vi "WPI_DashboardConvert to Log Format.vi"(11 "Frequent DB Data":T1) -> (3 "Logged Data":T2)   [LabVIEW 2017]
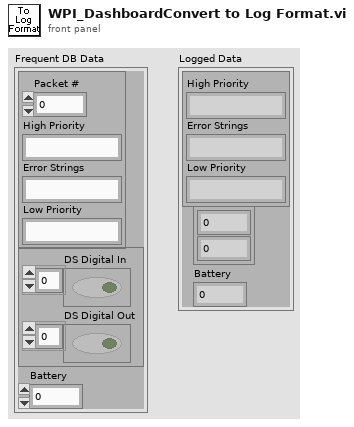
[diagram p1: front panel]
types:
  T1 = cluster{cluster{"Packet #":u8, "High Priority":string, "Error Strings":string, "Low Priority":string}, cluster{"DS Digital In":bool[], "DS Digital Out":bool[]}, "Battery":sgl}
  T2 = cluster{cluster{"High Priority":string, "Error Strings":string, "Low Priority":string}, cluster{u8, u8}, "Battery":sgl}
  T3 = cluster{"Packet #":u8, "High Priority":string, "Error Strings":string, "Low Priority":string}
  T4 = cluster{"DS Digital In":bool[], "DS Digital Out":bool[]}
  T5 = cluster{"High Priority":string, "Error Strings":string, "Low Priority":string}
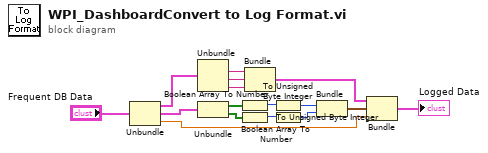
[diagram p0: block diagram]
diagram:
  n1 = Unbundle("Frequent DB Data") -> (w12:T3, w1:T4, "Battery"=w10:sgl)
  n2 = Unbundle(w12) -> ("High Priority"=w13:string, "Error Strings"=w15:string, "Low Priority"=w14:string)  [unwired: 1 out]
  n3 = Unbundle(w1) -> ("DS Digital In"=w2:bool[], "DS Digital Out"=w6:bool[])
  n4 = Boolean Array To Number(Boolean array=w2) -> (number=w3:u32)
  n5 = Boolean Array To Number(Boolean array=w6) -> (number=w5:u32)
  n6 = Bundle("High Priority"=w13, "Error Strings"=w15, "Low Priority"=w14) -> (w16:T5)  [unwired: 1 in]
  n7 = To Unsigned Byte Integer(number=w3) -> (unsigned 8bit integer=w4:u8)
  n8 = To Unsigned Byte Integer(number=w5) -> (unsigned 8bit integer=w7:u8)
  n9 = Bundle(w4, w7) -> (w9:cluster{u8, u8})  [unwired: 1 in]
  n10 = Bundle(w16, w9, "Battery"=w10) -> (→"Logged Data":T2)  [unwired: 1 in]
